vi "Template Match.vi"(6 "Match setup":T3={"Algorithm"=2, "Parameters"={"Number of Matches Requested"=1, "Minimum Match Score"=800.0, "Angle Ranges"=[]}, "Advanced Options"=[]} {"Algorithm" items=["All", "Low Discrepancy Sampling", "Grayscale Value Pyramid", "Gradients Pyramid"]; "Advanced Options"."Item" items=["LD Sampling - Minimum Constrast"=0, "LD Sampling - Enable Subpixel Accuracy"=1, "LD Sampling - Search Strategy"=2, "LD Sampling - Subpixel Iterations"=3, "LD Sampling - Subpixel Tolerance"=4, "LD Sampling - Initial Match List Length"=5, "LD Sampling - Match List Reduction Factor"=6, "LD Sampling - Initial Step Size"=7, "LD Sampling - Intermediate Angular Accuracy"=8, "-"=9, "Pyramid - Max Pyramid Level"=100, "Pyramid - Minimum Contrast"=102, "Pyramid - Enable Subpixel Accuracy"=103, "Pyramid - Subpixel Iterations"=104, "Pyramid - Subpixel Tolerance"=105, "Pyramid - Initial Match List Length"=106, "Pyramid - Match List Reduction Factor"=107, "Pyramid - Intermediate Angular Accuracy"=108, "Pyramid - Process Border Matches"=109, "Pyramid - Min Match Separation Distance"=111, "Pyramid - Min Match Separation Angle"=112, "Pyramid - Max Match Overlap"=113, "Pyramid - Max Cache in MB"=114, "Pyramid - Clear Cache"=115, "-"=116, "Enable Defect Map"=200]}, 8 "error in (no error)":errorcluster, 9 "ROI Descriptor":T4 {"Contours"."Type" items=["No Selection", "Point", "Line", "Rectangle", "Oval", "Polygon", "Freehand Region", "Annulus", "Unused2", "Unused3", "Broken Line", "Freehand Line", "Rotated Rectangle"]}, 10 "Template Image":T1, 11 "Image In":T1) -> (0 "error out":errorcluster, 1 "Matches (pixel)":T2(array[cluster]) {"Bounding Box"."y" format="%.2f"; "Bounding Box"."x" format="%.2f"; "Score" format="%.2f"; "Scale" format="%.2f"; "Angle" format="%.2f"; "Position"."y" format="%.2f"; "Position"."x" format="%.2f"}, 2 "Match?":bool, 3 "Image Out":T1)   [LabVIEW 2017]
uses:
  <vilib>/vision/Image Controls.llb/IMAQ Image.ctl
  <vilib>/vision/NI_Vision_Development_Module.lvlib
panel:
  out "Elapsed time(ms)":u32
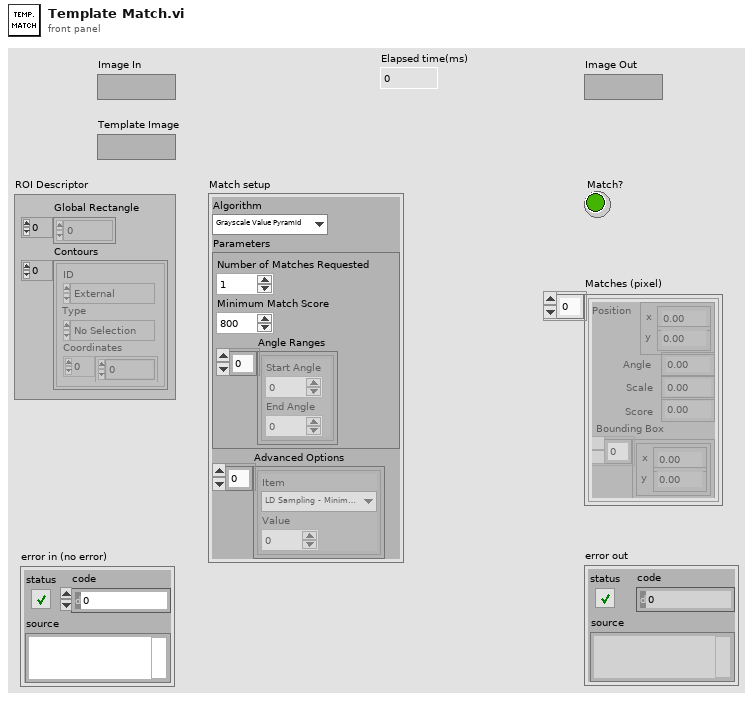
[diagram p1: front panel]
types:
  T1 = typedef "IMAQ Image.ctl" = refnum<image>
  T2 = cluster{"Position":cluster{"x":sgl, "y":sgl}, "Angle":sgl, "Scale":sgl, "Score":sgl, "Bounding Box":cluster{"x":sgl, "y":sgl}[]}[]
  T3 = cluster{"Algorithm":i32, "Parameters":cluster{"Number of Matches Requested":i32, "Minimum Match Score":sgl, "Angle Ranges":cluster{"Start Angle":sgl, "End Angle":sgl}[]}, "Advanced Options":cluster{"Item":u16, "Value":dbl}[]}
  T4 = typedef "ROI Descriptor" = cluster{"Global Rectangle":i32[], "Contours":cluster{"ID":enum32{"External", "Internal"}, "Type":u32, "Coordinates":i32[]}[]}
  T5 = cluster{"Number of Matches Requested":i32, "Minimum Match Score":sgl, "Angle Ranges":cluster{"Start Angle":sgl, "End Angle":sgl}[]}
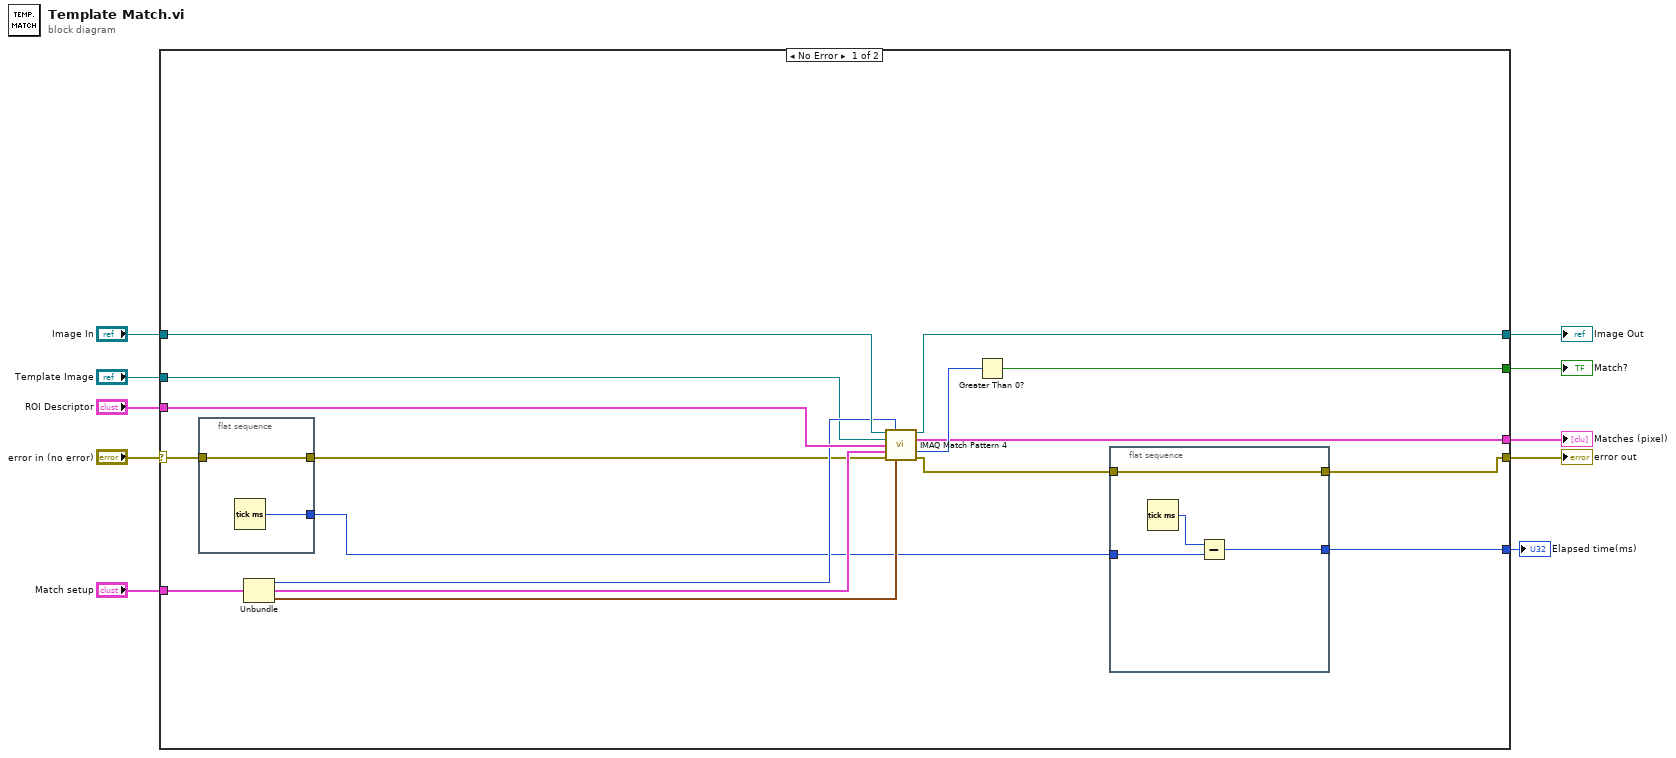
[diagram p0: block diagram]
diagram:
  n1 = case shown="No Error" "error in (no error)" {
    selector: "error in (no error)" -> [w16 w35]
    tunnel: [w15 w35] -> w9
    tunnel: "ROI Descriptor" -> [w26 _]
    tunnel: "Image In" -> [w25 w34]
    tunnel: "Match setup" -> [w24 _]
    tunnel: [w27 w34] -> w5
    tunnel: [w19 _] -> w4
    tunnel: [w18 _] -> w3
    tunnel: [w12 _] -> w2
    tunnel: "Template Image" -> [w11 _]
    frame No Error {
      n2 = flat-sequence {
        tunnel: [w33] -> w17
        tunnel: w16 -> [w33]
        tunnel: [w32] -> w13
        frame #0 {
          n3 = Tick Count (ms)() -> (millisecond timer value=w32:u32)
        }
      }
      n4 = Unbundle(w24) -> ("Algorithm"=w23:i32, "Parameters"=w22:T5, "Advanced Options"=w21:cluster{"Item":u16, "Value":dbl}[])
      n5 = call "IMAQ Match Pattern 4"("Image"=w25, "Algorithm"=w23, "Template Image"=w11, "ROI Descriptor"=w26, "Parameters"=w22, "error in (no error)"=w17, "Advanced Options"=w21) -> ("Image (duplicate)"=w27:T1, "Matches (pixel)"=w18:T2, "Number of Matches"=w20:i32, "error out"=w14:errorcluster)  [unwired: 4 in, 1 out]
      n6 = Greater Than 0?(x=w20) -> (x > 0?=w19:bool)
      n7 = flat-sequence {
        tunnel: [w31] -> w15
        tunnel: w14 -> [w31]
        tunnel: w13 -> [w29]
        tunnel: [w28] -> w12
        frame #0 {
          n8 = Tick Count (ms)() -> (millisecond timer value=w30:u32)
          n9 = Subtract(x=w30, y=w29) -> (x-y=w28:u32)
        }
      }
    }
    frame Error {
    }
  }
  "error out" <- w9
  "Image Out" <- w5
  "Match?" <- w4
  "Matches (pixel)" <- w3
  "Elapsed time(ms)" <- w2
